vi "Simulated Instrument Configurations.vi"(11 "Default Configuration":T1={"host IP (localhost)"="localhost", "host Port"=3388, "Model"="", "Serial Number(s)"="", "Calibration Date"=3388.0, "Dual Port?"=FALSE, "DeviceNames"=[], "Parameters"={"TX1start"=0.0, "TX1stop"=0.0, "TX1pmax"=0.0, "TX2start"=0.0, "TX2stop"=0.0, "TX2pmax"=0.0, "RXstart"=0.0, "RXstop"=0.0}, "Interface"=enum."PIM Web Engine"} {"Calibration Date" format="%.2f"; "Parameters"."TX2pmax" format="%.1f"; "Parameters"."TX1pmax" format="%.1f"; "Parameters"."RXstop" format="%.1f"; "Parameters"."RXstart" format="%.1f"; "Parameters"."TX2stop" format="%.1f"; "Parameters"."TX2start" format="%.1f"; "Parameters"."TX1stop" format="%.1f"; "Parameters"."TX1start" format="%.1f"}) -> (3 "Simulation Configurations":T1[](array[typedef])=[{"host IP (localhost)"="localhost", "host Port"=3388, "Model"="SI-1900", "Serial Number(s)"="1900D00000", "Calibration Date"=0.0, "Dual Port?"=TRUE, "DeviceNames"=["1900D00000-FE", "1823D00000-PA", "0727D00000-RF"], "Parameters"={"TX1start"=1930.0, "TX1stop"=1945.0, "TX1pmax"=48.0, "TX2start"=1960.0, "TX2stop"=1990.0, "TX2pmax"=48.0, "RXstart"=1850.0, "RXstop"=1910.0}, "Interface"=enum."PIM Web Engine"}, {"host IP (localhost)"="localhost", "host Port"=3388, "Model"="SI-800", "Serial Number(s)"="0800D00000", "Calibration Date"=0.0, "Dual Port?"=TRUE, "DeviceNames"=["0800D00000-FE", "0710D00000-PA", "0723D00000-RF"], "Parameters"={"TX1start"=869.0, "TX1stop"=871.6, "TX1pmax"=48.0, "TX2start"=889.0, "TX2stop"=894.0, "TX2pmax"=48.0, "RXstart"=824.0, "RXstop"=849.0}, "Interface"=enum."PIM Web Engine"}, {"host IP (localhost)"="localhost", "host Port"=3388, "Model"="SI-1800", "Serial Number(s)"="1800D00000", "Calibration Date"=0.0, "Dual Port?"=TRUE, "DeviceNames"=["1800D00000-FE", "1823D00000-PA", "0727D00000-RF"], "Parameters"={"TX1start"=1805.0, "TX1stop"=1820.0, "TX1pmax"=48.0, "TX2start"=1850.0, "TX2stop"=1880.0, "TX2pmax"=48.0, "RXstart"=1710.0, "RXstop"=1785.0}, "Interface"=enum."PIM Web Engine"}, {"host IP (localhost)"="localhost", "host Port"=3388, "Model"="SI-900", "Serial Number(s)"="0900D00000", "Calibration Date"=0.0, "Dual Port?"=TRUE, "DeviceNames"=["0900D00000-FE", "0710D00000-PA", "0727D00000-RF"], "Parameters"={"TX1start"=935.0, "TX1stop"=937.6, "TX1pmax"=48.0, "TX2start"=955.0, "TX2stop"=960.0, "TX2pmax"=48.0, "RXstart"=890.0, "RXstop"=915.0}, "Interface"=enum."PIM Web Engine"}, {"host IP (localhost)"="localhost", "host Port"=3388, "Model"="SI-2000", "Serial Number(s)"="2000D00000", "Calibration Date"=0.0, "Dual Port?"=TRUE, "DeviceNames"=["2000D00000-FE", "1823D00000-PA", "0727D00000-RF"], "Parameters"={"TX1start"=2110.0, "TX1stop"=2122.0, "TX1pmax"=48.0, "TX2start"=2153.0, "TX2stop"=2170.0, "TX2pmax"=48.0, "RXstart"=1920.0, "RXstop"=1980.0}, "Interface"=enum."PIM Web Engine"}] {"Calibration Date" format="%.2f"; "Parameters"."TX2pmax" format="%.1f"; "Parameters"."TX1pmax" format="%.1f"; "Parameters"."RXstop" format="%.1f"; "Parameters"."RXstart" format="%.1f"; "Parameters"."TX2stop" format="%.1f"; "Parameters"."TX2start" format="%.1f"; "Parameters"."TX1stop" format="%.1f"; "Parameters"."TX1start" format="%.1f"})   [LabVIEW 2011]
uses:
  PIM Configuration.ctl
  PIM Interface Language.ctl
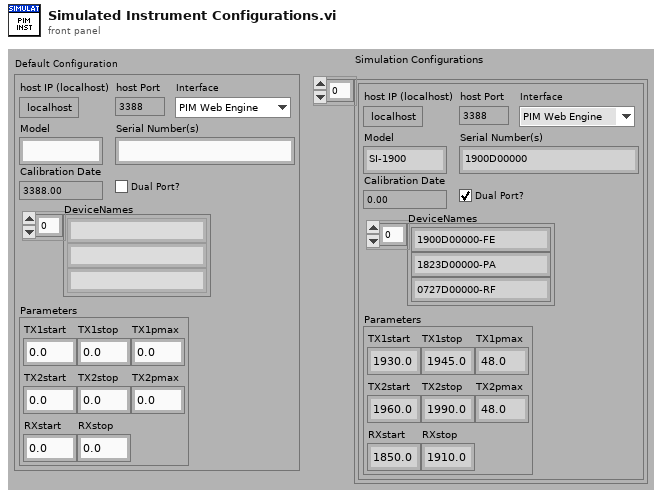
[diagram p1: front panel]
types:
  T1 = typedef "PIM Configuration.ctl" = cluster{"host IP (localhost)":string, "host Port":u16, "Model":string, "Serial Number(s)":string, "Calibration Date":dbl, "Dual Port?":bool, "DeviceNames":string[], "Parameters":cluster{"TX1start":dbl, "TX1stop":dbl, "TX1pmax":dbl, "TX2start":dbl, "TX2stop":dbl, "TX2pmax":dbl, "RXstart":dbl, "RXstop":dbl}, "Interface":T2}
  T2 = typedef "PIM Interface Language.ctl" = enum16{"PIM Web Engine", "PIM HW Engine"}
  T3 = enum16{"SI-700", "SI-800", "SI-900", "SI-1800", "SI-1900", "SI-2000", "SI-2600", "SI-3500"}[]
  T4 = cluster{"TX1start":dbl, "TX1stop":dbl, "TX1pmax":dbl, "TX2start":dbl, "TX2stop":dbl, "TX2pmax":dbl, "RXstart":dbl, "RXstop":dbl}
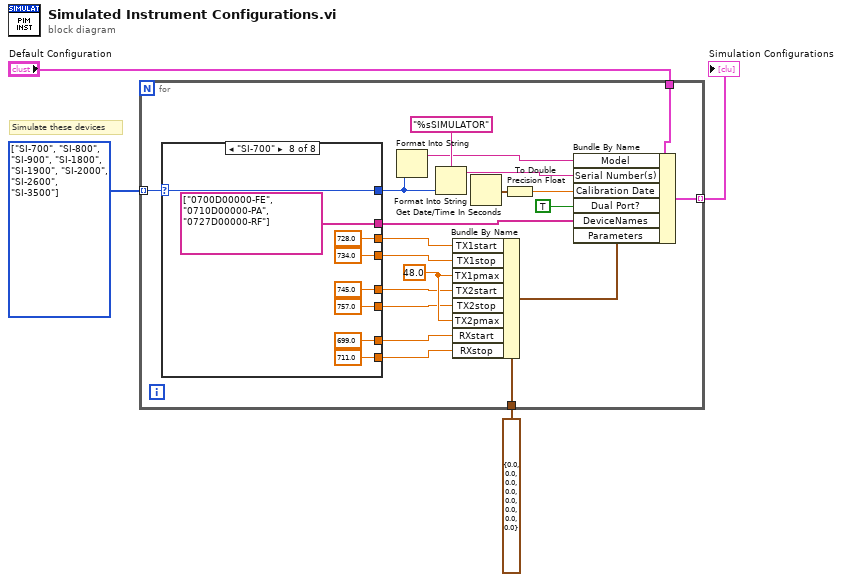
[diagram p0: block diagram]
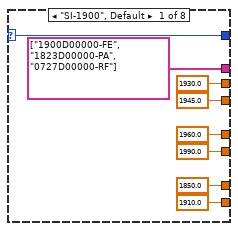
[diagram p2: hidden frame]
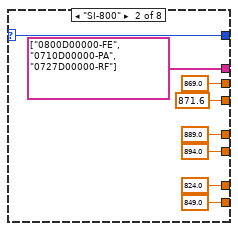
[diagram p3: hidden frame]
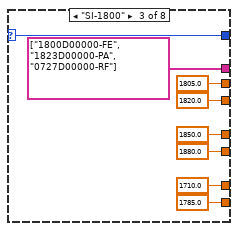
[diagram p4: hidden frame]
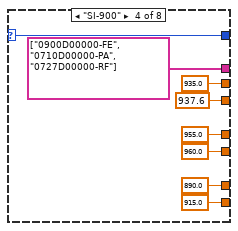
[diagram p5: hidden frame]
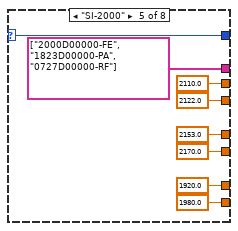
[diagram p6: hidden frame]
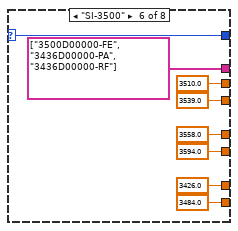
[diagram p7: hidden frame]
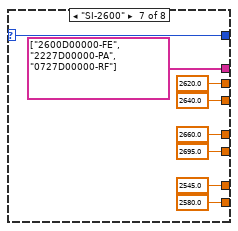
[diagram p8: hidden frame]
diagram:
  w2 = T3 [enum."SI-700", enum."SI-800", enum."SI-900", enum."SI-1800", enum."SI-1900", enum."SI-2000", enum."SI-2600", enum."SI-3500"] items=["SI-700", "SI-800", "SI-900", "SI-1800", "SI-1900", "SI-2000", "SI-2600", "SI-3500"]
  # "Simulate these devices"
  n1 = for {
    tunnel: T4 {"TX1start"=0.0, "TX1stop"=0.0, "TX1pmax"=0.0, "TX2start"=0.0, "TX2stop"=0.0, "TX2pmax"=0.0, "RXstart"=0.0, "RXstop"=0.0} ("Parameters") -> [w21]
    tunnel: "Default Configuration" -> [w7]
    tunnel: [w6] -> w1 mode=indexing
    tunnel: w2 -> [w5] mode=indexing
    w23 = 48.0 ("TX1pmax")
    n2 = case shown="\"SI-700\"" w5 {
      selector: w5 -> [w25 w33 w41 w49 w57 w65 w73 w81]
      tunnel: [1960.0 ("TX1start") 889.0 ("TX1start") 1850.0 ("TX1start") 955.0 ("TX1start") 2153.0 ("TX1start") 3558.0 ("TX1start") 2660.0 ("TX1start") 745.0 ("TX1start")] -> w20
      tunnel: [1990.0 ("TX1start") 894.0 ("TX1start") 1880.0 ("TX1start") 960.0 ("TX1start") 2170.0 ("TX1start") 3594.0 ("TX1start") 2695.0 ("TX1start") 757.0 ("TX1start")] -> w19
      tunnel: [1930.0 ("TX1start") 869.0 ("TX1start") 1805.0 ("TX1start") 935.0 ("TX1start") 2110.0 ("TX1start") 3510.0 ("TX1start") 2620.0 ("TX1start") 728.0 ("TX1start")] -> w18
      tunnel: [1945.0 ("TX1start") 871.6 ("TX1start") 1820.0 ("TX1start") 937.6 ("TX1start") 2122.0 ("TX1start") 3539.0 ("TX1start") 2640.0 ("TX1start") 734.0 ("TX1start")] -> w17
      tunnel: [1910.0 ("TX1start") 849.0 ("TX1start") 1785.0 ("TX1start") 915.0 ("TX1start") 1980.0 ("TX1start") 3484.0 ("TX1start") 2580.0 ("TX1start") 711.0 ("TX1start")] -> w16
      tunnel: [1850.0 ("TX1start") 824.0 ("TX1start") 1710.0 ("TX1start") 890.0 ("TX1start") 1920.0 ("TX1start") 3426.0 ("TX1start") 2545.0 ("TX1start") 699.0 ("TX1start")] -> w15
      tunnel: [string[] ["1900D00000-FE", "1823D00000-PA", "0727D00000-RF"] ("DeviceNames") string[] ["0800D00000-FE", "0710D00000-PA", "0727D00000-RF"] ("DeviceNames") string[] ["1800D00000-FE", "1823D00000-PA", "0727D00000-RF"] ("DeviceNames") string[] ["0900D00000-FE", "0710D00000-PA", "0727D00000-RF"] ("DeviceNames") string[] ["2000D00000-FE", "1823D00000-PA", "0727D00000-RF"] ("DeviceNames") string[] ["3500D00000-FE", "3436D00000-PA", "3436D00000-RF"] ("DeviceNames") string[] ["2600D00000-FE", "2227D00000-PA", "0727D00000-RF"] ("DeviceNames") string[] ["0700D00000-FE", "0710D00000-PA", "0727D00000-RF"] ("DeviceNames")] -> w14
      tunnel: [w25 w33 w41 w49 w57 w65 w73 w81] -> w9
      frame "SI-1900", Default {
      }
      frame "SI-800" {
      }
      frame "SI-1800" {
      }
      frame "SI-900" {
      }
      frame "SI-2000" {
      }
      frame "SI-3500" {
      }
      frame "SI-2600" {
      }
      frame "SI-700" {
      }
    }
    n3 = Format Into String(w9) -> (resulting string=w10:string)  [unwired: 3 in, 1 out]
    n4 = Format Into String(format string="%sSIMULATOR", w9) -> (resulting string=w11:string)  [unwired: 2 in, 1 out]
    n5 = Bundle By Name(cluster=w21, "TX1start"=w18, "TX1stop"=w17, "TX1pmax"=w23, "TX2start"=w20, "TX2stop"=w19, "TX2pmax"=w23, "RXstart"=w15, "RXstop"=w16) -> (w22:T4)
    n6 = Get Date/Time In Seconds() -> (seconds since 1Jan1904=w24:timestamp)
    n7 = To Double Precision Float(number=w24) -> (double precision float=w8:dbl)
    n8 = Bundle By Name(cluster=w7, "Model"=w10, "Serial Number(s)"=w11, "Calibration Date"=w8, "Dual Port?"=TRUE, "DeviceNames"=w14, "Parameters"=w22) -> (w6:T1)
  }
  "Simulation Configurations" <- w1
